vi "Daemon.vi"(8 "error in (no error)":errorcluster, 11 "WAMP Client in":refnum<class "WAMP Client.lvclass">) -> (0 "error out":errorcluster, 3 "WAMP Client out":refnum<class "WAMP Client.lvclass">)   [LabVIEW 2021, in "wamplv.lvlib" / "WAMP Client.lvclass"]
uses:
  WAMP Client.lvclass
  WAMP Client.lvclass/WAMP Client.ctl
  Private/Comm Handlers/ICommHandler/ICommHandler.lvclass
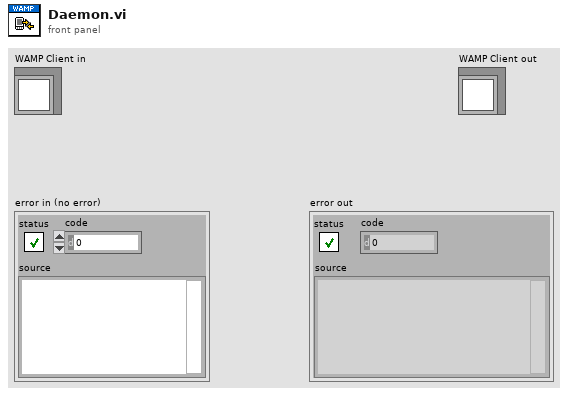
[diagram p1: front panel]
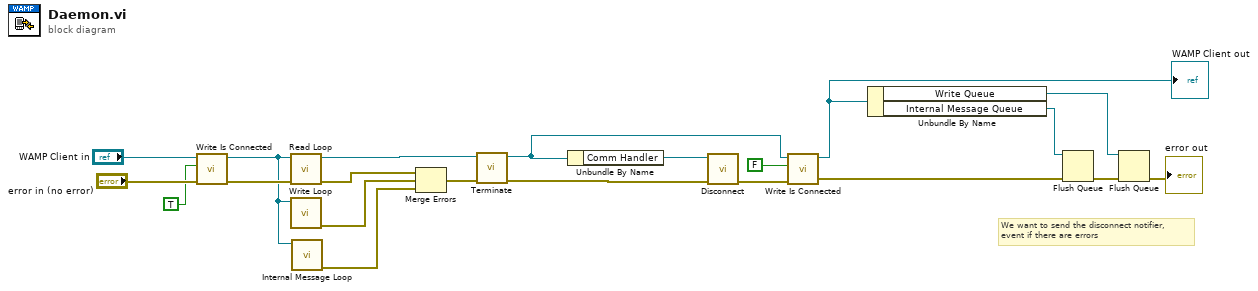
[diagram p0: block diagram]
diagram:
  # "We want to send the disconnect notifier,\nevent if there are errors"
  n1 = call "Write Is Connected.vi"("error in (no error)"="error in (no error)", "Connected?"=TRUE, "WAMP Client in"="WAMP Client in") -> ("error out"=w5:errorcluster, "WAMP Client out"=w4:refnum<class "WAMP Client.lvclass">)  [unwired: 7 in]
  n2 = call-dynamic "Read Loop.vi"("error in (no error)"=w5, "WAMP Client in"=w4) -> ("error out"=w13:errorcluster, "WAMP Client out"=w10:refnum<class "WAMP Client.lvclass">)  [unwired: 8 in]
  n3 = call-dynamic "Write Loop.vi"("WAMP Client in"=w4) -> ("error out"=w12:errorcluster)  [unwired: 9 in, 1 out]
  n4 = call-dynamic "Internal Message Loop.vi"("WAMP Client in"=w4) -> ("error out"=w11:errorcluster)  [unwired: 9 in, 1 out]
  n5 = Merge Errors(w13, w12, w11) -> (w9:errorcluster)
  n6 = call-dynamic "Terminate.vi"("error in (no error)"=w9, "WAMP Client in"=w10) -> ("error out"=w7:errorcluster, "WAMP Client out"=w14:refnum<class "WAMP Client.lvclass">)  [unwired: 8 in]
  n7 = Unbundle By Name(w14) -> ("Comm Handler"=w15:refnum<class "ICommHandler.lvclass">)
  n8 = call-dynamic "Disconnect.vi"("error in (no error)"=w7, "ICommHandler in"=w15) -> ("error out"=w6:errorcluster)  [unwired: 8 in, 1 out]
  n9 = call "Write Is Connected.vi"("error in (no error)"=w6, "Connected?"=FALSE ("data value"), "WAMP Client in"=w14) -> ("error out"=w17:errorcluster, "WAMP Client out"=w18:refnum<class "WAMP Client.lvclass">)  [unwired: 7 in]
  "WAMP Client out" <- w18
  n10 = Unbundle By Name(w18) -> ("Write Queue"=w19:refnum<queue>, "Internal Message Queue"=w20:refnum<queue>)
  n11 = Flush Queue(queue=w20, error in (no error)=w17) -> (error out=w21:errorcluster)  [unwired: 2 out]
  n12 = Flush Queue(queue=w19, error in (no error)=w21) -> (error out=→"error out":errorcluster)  [unwired: 2 out]
